vi "LoadApplicationConfig.vi"(8 "error in (no error)":errorcluster) -> (0 "error out":errorcluster, 2 "Config Cluster":T1, 3 "refnum out":T5)   [LabVIEW 2026]
uses:
  <vilib>/Utility/config.llb/Config Data RefNum.ctl
  controls/Vibration_Monitor_Config.ctl
  controls/Vibration_Profile.ctl
  controls/System_Settings.ctl
  controls/Options.ctl
  <vilib>/Utility/config.llb/Read Key (String).vi
  <vilib>/Utility/config.llb/Read Key (I32).vi
  <vilib>/Utility/config.llb/Read Key (Double).vi
  <vilib>/Utility/config.llb/NI_LVConfig.lvlib
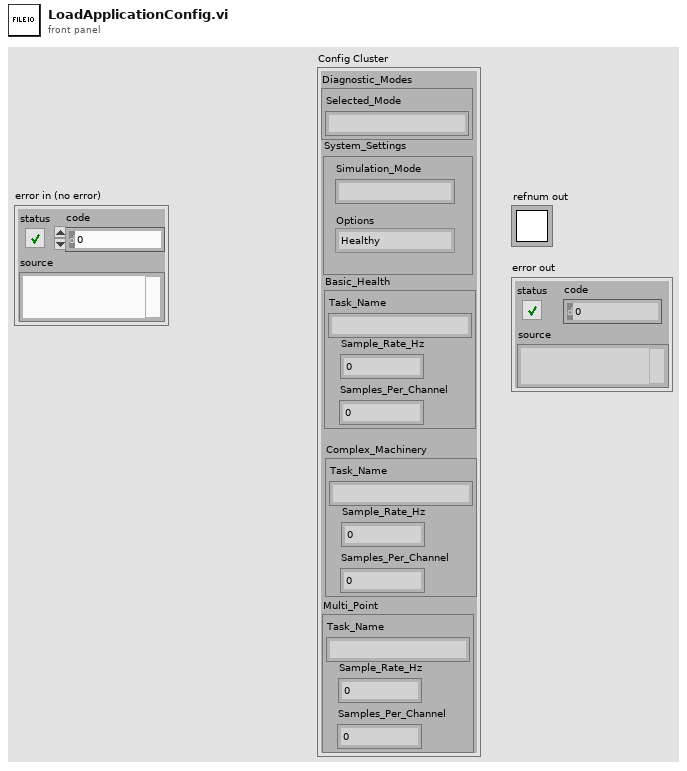
[diagram p1: front panel]
types:
  T1 = typedef "Vibration_Monitor_Config.ctl" = cluster{"Diagnostic_Modes":cluster{"Selected_Mode":string}, "Basic_Health":T2, "Complex_Machinery":T2, "Multi_Point":T2, "System_Settings":T3}
  T2 = typedef "Vibration_Profile.ctl" = cluster{"Task_Name":string, "Sample_Rate_Hz":dbl, "Samples_Per_Channel":i32}
  T3 = typedef "System_Settings.ctl" = cluster{"Simulation_Mode ":string, "Options":T4}
  T4 = typedef "Options.ctl" = enum16{"Healthy", "Unbalance_Alert", "Bearing_Fault_Critical", "Sweep_Test"}
  T5 = typedef "NI_LVConfig.lvlib/Config Data RefNum.ctl" = refnum<k1>
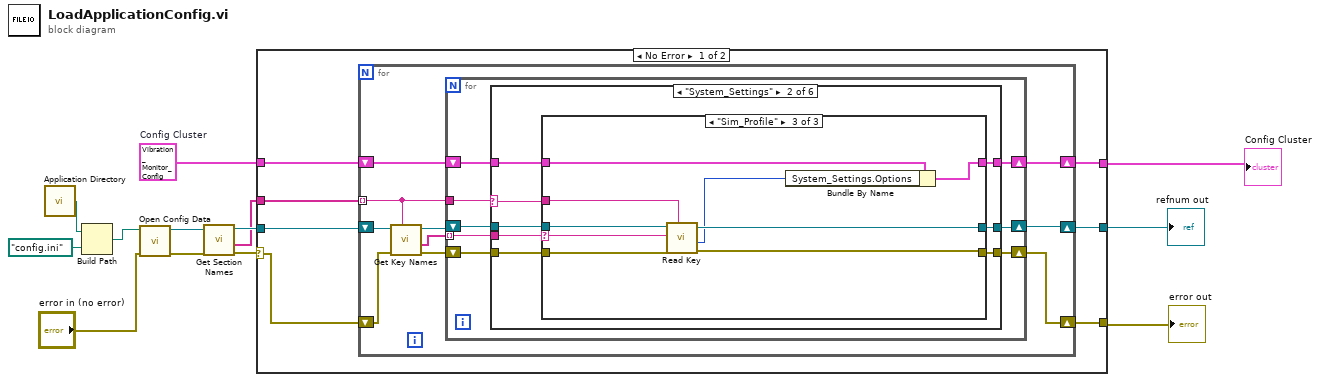
[diagram p0: block diagram]
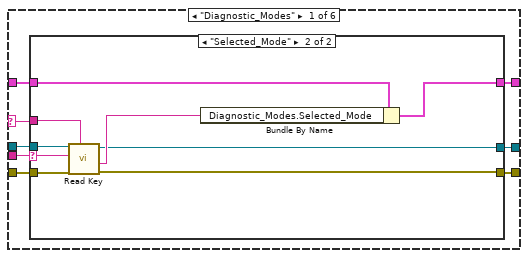
[diagram p2: hidden frame]
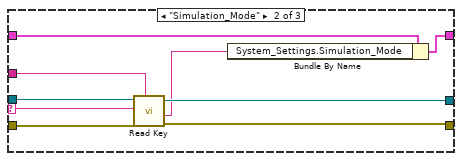
[diagram p5: hidden frame]
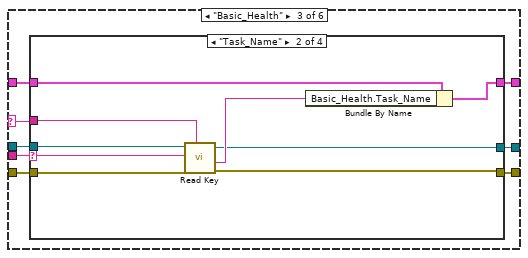
[diagram p6: hidden frame]
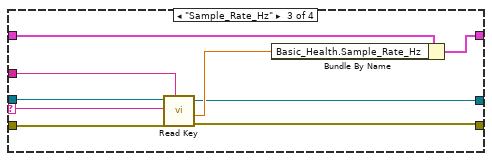
[diagram p8: hidden frame]
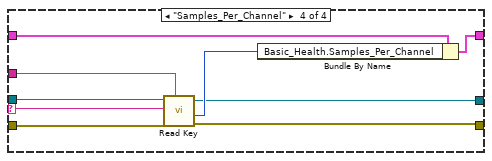
[diagram p9: hidden frame]
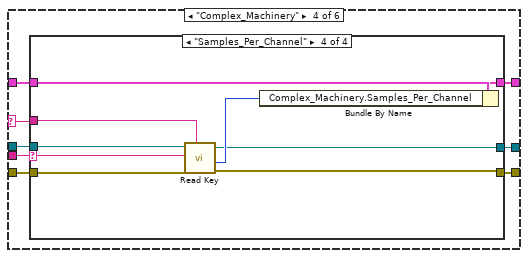
[diagram p10: hidden frame]
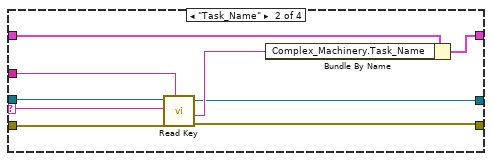
[diagram p12: hidden frame]
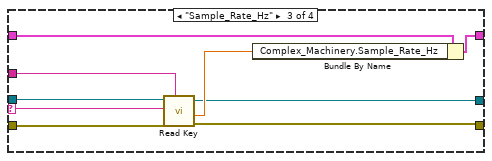
[diagram p13: hidden frame]
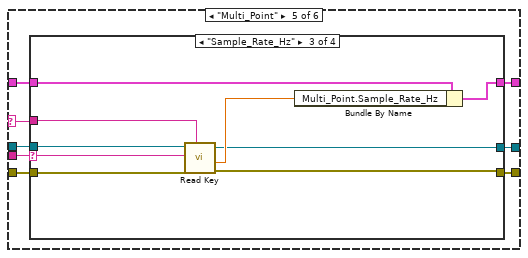
[diagram p14: hidden frame]
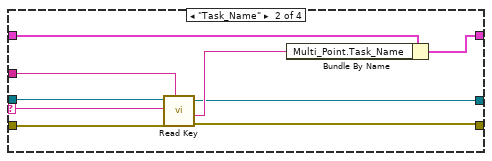
[diagram p16: hidden frame]
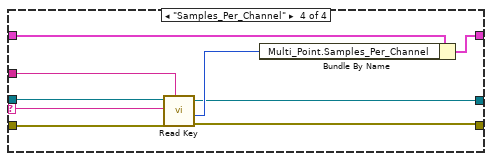
[diagram p17: hidden frame]
diagram:
  w2 = T1 {"Diagnostic_Modes"={"Selected_Mode"=""}, "Basic_Health"={"Task_Name"="", "Sample_Rate_Hz"=0.0, "Samples_Per_Channel"=0}, "Complex_Machinery"={"Task_Name"="", "Sample_Rate_Hz"=0.0, "Samples_Per_Channel"=0}, "Multi_Point"={"Task_Name"="", "Sample_Rate_Hz"=0.0, "Samples_Per_Channel"=0}, "System_Settings"={"Simulation_Mode "="", "Options"=enum."Healthy"}}  # Config Cluster
  n1 = call <vilib>:"Application Directory.vi"() -> ("Application Directory"=w12:path)
  n2 = Build Path(base path=w12, name or relative path=path "config.ini") -> (appended path=w13:path)
  n3 = call <vilib>:"Open Config Data.vi"("error in (no error)"="error in (no error)", "configuration file path"=w13) -> ("error out"=w9:errorcluster, "refnum"=w10:T5)  [unwired: 7 in, 1 out]
  n4 = call <vilib>:"Get Section Names.vi"("error in (no error)"=w9, "refnum"=w10) -> ("error out"=w6:errorcluster, "section names"=w4:string[], "refnum out"=w5:T5)  [unwired: 7 in]
  n5 = case shown="No Error" w6 {
    selector: w6 -> [w19 w207]
    tunnel: [w17 w207] -> w8
    tunnel: w5 -> [w20 w206]
    tunnel: w4 -> [w18 _]
    tunnel: [w16 w206] -> w3
    tunnel: w2 -> [w15 w205]
    tunnel: [w14 w205] -> w1
    frame No Error {
      n6 = for {
        tunnel: w18 -> [w21] mode=indexing
        shift-right: [w26] -> w17
        shift-left: w19 -> [w29]
        shift-right: [w24] -> w16
        shift-left: w20 -> [w30]
        shift-right: [w22] -> w14
        shift-left: w15 -> [w23]
        n7 = call <vilib>:"Get Key Names.vi"("section"=w21, "error in (no error)"=w29, "refnum"=w30) -> ("error out"=w28:errorcluster, "key names"=w25:string[], "refnum out"=w27:T5)  [unwired: 5 in, 1 out]
        n8 = for {
          shift-right: [w33] -> w26
          shift-left: w28 -> [w35]
          tunnel: w25 -> [w36] mode=indexing
          shift-right: [w32] -> w24
          shift-left: w27 -> [w34]
          shift-right: [w38] -> w22
          shift-left: w23 -> [w37]
          tunnel: w21 -> [w31]
          n9 = case shown="\"System_Settings\"" w31 {
            selector: w31 -> [w39 w59 w88 w126 w164 _]
            tunnel: [w46 w66 w95 w133 w171 w204] -> w38
            tunnel: w37 -> [w45 w65 w94 w132 w170 w204]
            tunnel: w36 -> [w44 w64 w93 w131 w169 _]
            tunnel: w35 -> [w43 w63 w92 w130 w168 w202]
            tunnel: w34 -> [w42 w62 w91 w129 w167 w203]
            tunnel: [w41 w61 w90 w128 w166 w202] -> w33
            tunnel: [w40 w60 w89 w127 w165 w203] -> w32
            frame "Diagnostic_Modes" {
              n10 = case shown="\"Selected_Mode\"" w44 {
                selector: w44 -> [_ w57]
                tunnel: [w49 w56] -> w46
                tunnel: w45 -> [w49 w58]
                tunnel: w39 -> [_ w55]
                tunnel: w43 -> [w48 w53]
                tunnel: w42 -> [w47 w52]
                tunnel: [w48 w51] -> w41
                tunnel: [w47 w50] -> w40
                frame Default {
                }
                frame "Selected_Mode" {
                  n11 = call-poly <vilib>:"Read Key.vi"("section"=w55, "error in (no error)"=w53, "key"=w57, "refnum"=w52) -> ("error out"=w51:errorcluster, "value"=w54:string, "refnum out"=w50:T5)  [unwired: 4 in, 1 out]
                  n12 = Bundle By Name(cluster=w58, "Diagnostic_Modes.Selected_Mode"=w54) -> (w56:T1)
                }
              }
            }
            frame "System_Settings" {
              n13 = case shown="\"Sim_Profile\"" w64 {
                selector: w64 -> [_ w73 w82]
                tunnel: [w69 w77 w86] -> w66
                tunnel: w65 -> [w69 w78 w87]
                tunnel: w59 -> [_ w74 w83]
                tunnel: w63 -> [w67 w75 w84]
                tunnel: w62 -> [w68 w76 w85]
                tunnel: [w67 w72 w81] -> w61
                tunnel: [w68 w71 w80] -> w60
                frame Default {
                }
                frame "Simulation_Mode" {
                  n14 = call-poly <vilib>:"Read Key.vi"("section"=w74, "error in (no error)"=w75, "key"=w73, "refnum"=w76) -> ("error out"=w72:errorcluster, "value"=w70:string, "refnum out"=w71:T5)  [unwired: 4 in, 1 out]
                  n15 = Bundle By Name(cluster=w78, "System_Settings.Simulation_Mode"=w70) -> (w77:T1)
                }
                frame "Sim_Profile" {
                  n16 = call-poly <vilib>:"Read Key.vi"("section"=w83, "error in (no error)"=w84, "key"=w82, "refnum"=w85) -> ("error out"=w81:errorcluster, "value"=w79:i32, "refnum out"=w80:T5)  [unwired: 4 in, 1 out]
                  n17 = Bundle By Name(cluster=w87, "System_Settings.Options"=w79) -> (w86:T1)
                }
              }
            }
            frame "Basic_Health" {
              n18 = case shown="\"Task_Name\"" w93 {
                selector: w93 -> [_ w101 w110 w119]
                tunnel: [w98 w106 w115 w124] -> w95
                tunnel: w94 -> [w98 w107 w116 w125]
                tunnel: w88 -> [_ w103 w112 w121]
                tunnel: w92 -> [w96 w104 w113 w122]
                tunnel: w91 -> [w97 w105 w114 w123]
                tunnel: [w96 w100 w109 w118] -> w90
                tunnel: [w97 w99 w108 w117] -> w89
                frame Default {
                }
                frame "Task_Name" {
                  n19 = call-poly <vilib>:"Read Key.vi"("section"=w103, "error in (no error)"=w104, "key"=w101, "refnum"=w105) -> ("error out"=w100:errorcluster, "value"=w102:string, "refnum out"=w99:T5)  [unwired: 4 in, 1 out]
                  n20 = Bundle By Name(cluster=w107, "Basic_Health.Task_Name"=w102) -> (w106:T1)
                }
                frame "Sample_Rate_Hz" {
                  n21 = call-poly <vilib>:"Read Key.vi"("section"=w112, "error in (no error)"=w113, "key"=w110, "refnum"=w114) -> ("error out"=w109:errorcluster, "value"=w111:dbl, "refnum out"=w108:T5)  [unwired: 4 in, 1 out]
                  n22 = Bundle By Name(cluster=w116, "Basic_Health.Sample_Rate_Hz"=w111) -> (w115:T1)
                }
                frame "Samples_Per_Channel" {
                  n23 = call-poly <vilib>:"Read Key.vi"("section"=w121, "error in (no error)"=w122, "key"=w119, "refnum"=w123) -> ("error out"=w118:errorcluster, "value"=w120:i32, "refnum out"=w117:T5)  [unwired: 4 in, 1 out]
                  n24 = Bundle By Name(cluster=w125, "Basic_Health.Samples_Per_Channel"=w120) -> (w124:T1)
                }
              }
            }
            frame "Complex_Machinery" {
              n25 = case shown="\"Samples_Per_Channel\"" w131 {
                selector: w131 -> [_ w139 w148 w157]
                tunnel: [w136 w144 w153 w162] -> w133
                tunnel: w132 -> [w136 w145 w154 w163]
                tunnel: w126 -> [_ w141 w150 w159]
                tunnel: w130 -> [w134 w142 w151 w160]
                tunnel: w129 -> [w135 w143 w152 w161]
                tunnel: [w134 w138 w147 w156] -> w128
                tunnel: [w135 w137 w146 w155] -> w127
                frame Default {
                }
                frame "Task_Name" {
                  n26 = call-poly <vilib>:"Read Key.vi"("section"=w141, "error in (no error)"=w142, "key"=w139, "refnum"=w143) -> ("error out"=w138:errorcluster, "value"=w140:string, "refnum out"=w137:T5)  [unwired: 4 in, 1 out]
                  n27 = Bundle By Name(cluster=w145, "Complex_Machinery.Task_Name"=w140) -> (w144:T1)
                }
                frame "Sample_Rate_Hz" {
                  n28 = call-poly <vilib>:"Read Key.vi"("section"=w150, "error in (no error)"=w151, "key"=w148, "refnum"=w152) -> ("error out"=w147:errorcluster, "value"=w149:dbl, "refnum out"=w146:T5)  [unwired: 4 in, 1 out]
                  n29 = Bundle By Name(cluster=w154, "Complex_Machinery.Sample_Rate_Hz"=w149) -> (w153:T1)
                }
                frame "Samples_Per_Channel" {
                  n30 = call-poly <vilib>:"Read Key.vi"("section"=w159, "error in (no error)"=w160, "key"=w157, "refnum"=w161) -> ("error out"=w156:errorcluster, "value"=w158:i32, "refnum out"=w155:T5)  [unwired: 4 in, 1 out]
                  n31 = Bundle By Name(cluster=w163, "Complex_Machinery.Samples_Per_Channel"=w158) -> (w162:T1)
                }
              }
            }
            frame "Multi_Point" {
              n32 = case shown="\"Sample_Rate_Hz\"" w169 {
                selector: w169 -> [_ w177 w186 w195]
                tunnel: [w174 w182 w191 w200] -> w171
                tunnel: w170 -> [w174 w183 w192 w201]
                tunnel: w164 -> [_ w179 w188 w197]
                tunnel: w168 -> [w172 w180 w189 w198]
                tunnel: w167 -> [w173 w181 w190 w199]
                tunnel: [w172 w176 w185 w194] -> w166
                tunnel: [w173 w175 w184 w193] -> w165
                frame Default {
                }
                frame "Task_Name" {
                  n33 = call-poly <vilib>:"Read Key.vi"("section"=w179, "error in (no error)"=w180, "key"=w177, "refnum"=w181) -> ("error out"=w176:errorcluster, "value"=w178:string, "refnum out"=w175:T5)  [unwired: 4 in, 1 out]
                  n34 = Bundle By Name(cluster=w183, "Multi_Point.Task_Name"=w178) -> (w182:T1)
                }
                frame "Sample_Rate_Hz" {
                  n35 = call-poly <vilib>:"Read Key.vi"("section"=w188, "error in (no error)"=w189, "key"=w186, "refnum"=w190) -> ("error out"=w185:errorcluster, "value"=w187:dbl, "refnum out"=w184:T5)  [unwired: 4 in, 1 out]
                  n36 = Bundle By Name(cluster=w192, "Multi_Point.Sample_Rate_Hz"=w187) -> (w191:T1)
                }
                frame "Samples_Per_Channel" {
                  n37 = call-poly <vilib>:"Read Key.vi"("section"=w197, "error in (no error)"=w198, "key"=w195, "refnum"=w199) -> ("error out"=w194:errorcluster, "value"=w196:i32, "refnum out"=w193:T5)  [unwired: 4 in, 1 out]
                  n38 = Bundle By Name(cluster=w201, "Multi_Point.Samples_Per_Channel"=w196) -> (w200:T1)
                }
              }
            }
            frame Default {
            }
          }
        }
      }
    }
    frame Error {
    }
  }
  "error out" <- w8
  "refnum out" <- w3
  "Config Cluster" <- w1
